vi "Set Relay Control.vi"(7 "state handshake":T2, 10 "stream.state":T1, 11 "samples transferred":u64) -> (4 "ready for input":bool)   [LabVIEW 2015, in "niInstr Streaming v1 FPGA.lvlib"]
uses:
  <instrlib>/_niInstr/Streaming/v1/FPGA/niInstr Streaming v1 FPGA.lvlib
  <instrlib>/_niInstr/Streaming/v1/FPGA/Public/Stream Additive Count Register.ctl
  <instrlib>/_niInstr/Streaming/v1/Common/Stream State.ctl
  <instrlib>/_niInstr/Streaming/v1/FPGA/Public/Stream Additive Count Data.ctl
  <vilib>/rvi/Emulation/niFpgaSctlEmulationGetInTimedLoop.vi
  <vilib>/rvi/DataTransferAndStorage/Container/Common/niFpgaContainerExecOnDevCompGetState.vi
  <vilib>/rvi/Emulation/niFpgaEmulationIsFPGAContextNoSignature.vi
  <vilib>/rvi/DataTransferAndStorage/Container/Common/niFpgaContainerGetUniqueNameForEmu.vi
  <vilib>/rvi/eio/common/nirviEmuReportErrorAndStop.vi
  <vilib>/rvi/Emulation/niFpgaProcessEmulError.vi
  <vilib>/rvi/DataTransferAndStorage/Container/XNode/niFpgaContainer.xnode
  <vilib>/rvi/DataTransferAndStorage/Handshake/Emulation/niFpgaHandshakeEmulationRefIn.vi
  <instrlib>/_niInstr/Streaming/v1/Common/niInstr Streaming v1 Common.lvlib
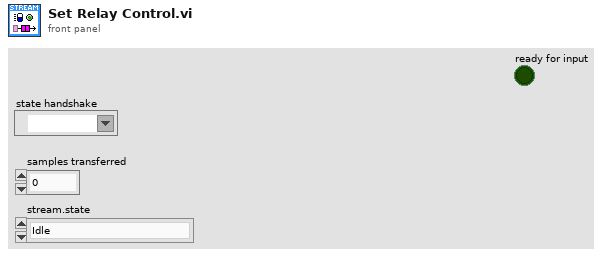
[diagram p1: front panel]
types:
  T1 = typedef "niInstr Streaming v1 Common.lvlib/Stream State.ctl" = enum8{"Idle", "Finite Transfer", "Continuous", "Done", "Error", "Not Ready", "Cancel"}
  T2 = typedef "niInstr Streaming v1 FPGA.lvlib/Stream Additive Count Register.ctl" = refnum<k21>
  T3 = typedef "niInstr Streaming v1 FPGA.lvlib/Stream Additive Count Data.ctl" = cluster{"stream.state":T1, "stream.additive num samples":u16}
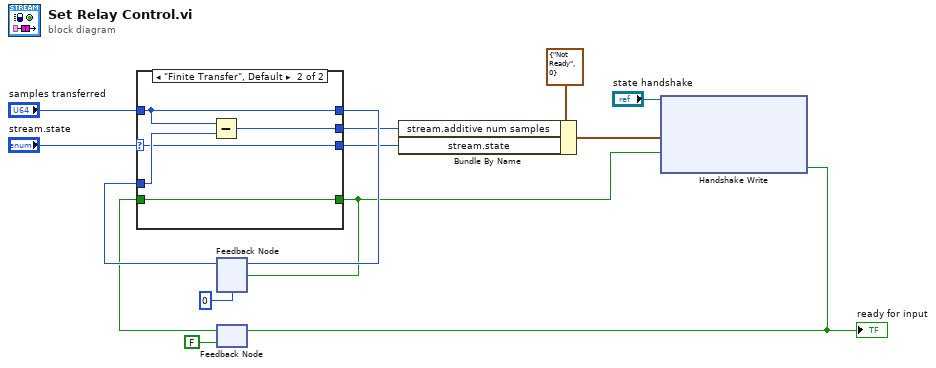
[diagram p0: block diagram]
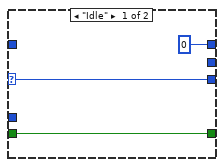
[diagram p2: hidden frame]
diagram:
  n1 = feedback #1(u64 0 ("samples transferred")) -> (w8:u64)
  n2 = feedback #2(FALSE ("Ready for Input")) -> (w6:bool)
  n3 = case shown="\"Finite Transfer\", Default" "stream.state" {
    selector: "stream.state" -> [w16 w18]
    tunnel: "samples transferred" -> [_ w19]
    tunnel: [u64 0 ("samples transferred") w19] -> w9
    tunnel: w8 -> [_ w22]
    tunnel: w6 -> [w17 w20]
    tunnel: [w17 w20] -> w3
    tunnel: [w16 w18] -> w1
    tunnel: [_ w21] -> w2
    frame "Idle" {
    }
    frame "Finite Transfer", Default {
      n4 = Subtract(x=w19, y=w22) -> (x-y=w21:u64)
    }
  }
  n5 = feedback-in #1(w9, w3) -> ()
  n6 = Bundle By Name(cluster=T3 {"stream.state"=enum."Not Ready", "stream.additive num samples"=0} ("Cluster"), "stream.additive num samples"=w2, "stream.state"=w1) -> (w4:T3)
  n7 = xnode ("Handshake Write")("Data"=w4, "Input Valid"=w3, "Handshake In"="state handshake") -> ("Ready for Input"=w13:bool)  [unwired: 1 out]
  "ready for input" <- w13
  n8 = feedback-in #2(w13) -> ()
